vi "Cross Power (CDB).vi"(2 "Y":cdb[](array[numeric]), 3 "X":cdb[](array[numeric])) -> (0 "error":i32, 1 "Sxy":cdb[](array[numeric]))   [LabVIEW 2014, in "NI_AALPro.lvlib"]
doc: "Computes the cross power spectrum, <B>Sxy</B>, of the input signals <B>X</B> and <B>Y</B>. Wire data to the <B>X</B> input to determine the polymorphic instance to use or manually select the instance."
uses:
  NI_AALPro.lvlib
  lvanlys.dll
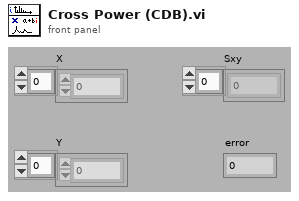
[diagram p1: front panel]
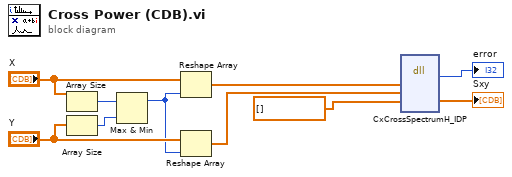
[diagram p0: block diagram]
diagram:
  n1 = Array Size(array="X") -> (size(s)=w6:i32)
  n2 = Array Size(array="Y") -> (size(s)=w5:i32)
  n3 = Max & Min(x=w6, y=w5) -> (max(x,y)=w4:i32)  [unwired: 1 out]
  n4 = Reshape Array("X", w4) -> (w7:cdb[])
  n5 = Reshape Array("Y", w4) -> (w8:cdb[])
  n6 = dll-call lib="C:/Program Files (x86)/National Instruments/LabVIEW 2014/resource/lvanlys.*" fn="CxCrossSpectrumH_IDP"("xH"=w7, "yH"=w8, "zH"=cdb[] [] ("Sxy")) -> ("return type"=→"error":i32, "zH"=→"Sxy":cdb[])  [unwired: 7 in, 2 out]
